vi "Purge.vi"(5 "Digital I/O Pin":u8=7, 7 "Arduino Resource":T1={"VISA resource"="GlueCTRL", "Board Type"=enum."Uno", "Connection Type"=enum."USB / Serial", "Bytes Per Packet (15)"=15}, 8 "Purge Time [ms]":dbl format="%#_13g", 9 "Axis Speeds":T3={"X [mm/s]"=25.0, "Y [mm/s]"=25.0, "Z [mm/s]"=25.0}, 10 "Start Position [mm]":dbl[](array[numeric]), 11 ".NET Refnum In":refnum<k24>) -> ()   [LabVIEW 2016]
uses:
  C:/Users/Aerotech/Documents/BNLStaveAssembly-blueprint/Bin/Aerotech.A3200.dll
  BNLStaveAssembly-blueprint/Bin/Aerotech.A3200.dll
  <vilib>/LabVIEW Interface for Arduino/Type Defs/Arduino Resource.ctl
  <vilib>/LabVIEW Interface for Arduino/Type Defs/Board Type.ctl
  <vilib>/LabVIEW Interface for Arduino/LabVIEW Interface for Arduino.lvlib
panel:
  in  "Change to Purge [mm]":dbl[](array[numeric])=[0.0, -15.0, 0.0]
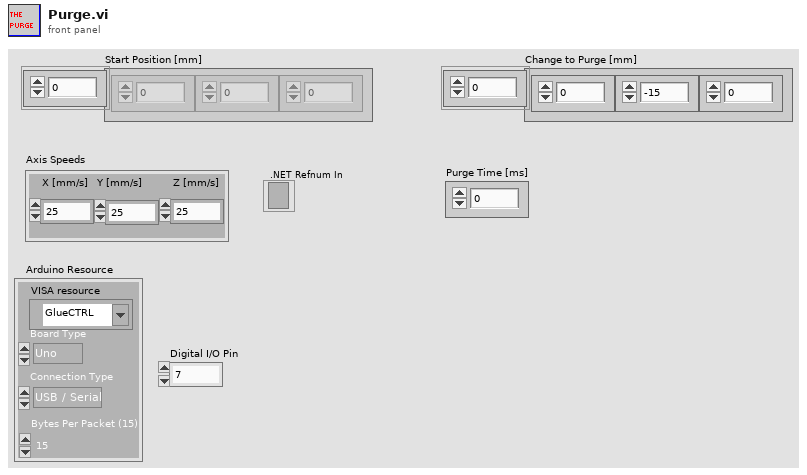
[diagram p1: front panel]
types:
  T1 = typedef "LabVIEW Interface for Arduino.lvlib/Arduino Resource.ctl" = cluster{"VISA resource":refnum<visa-resource-name>, "Board Type":T2, "Connection Type":enum8{"USB / Serial"}, "Bytes Per Packet (15)":u8}
  T2 = typedef "LabVIEW Interface for Arduino.lvlib/Board Type.ctl" = enum16{"Uno", "Dimuelanove w/Atmega 328", "Mega 2560"}
  T3 = cluster{"X [mm/s]":dbl, "Y [mm/s]":dbl, "Z [mm/s]":dbl}
  T4 = cluster{"Start Position [mm][0]":dbl, "Start Position [mm][1]":dbl, "Start Position [mm][2]":dbl}
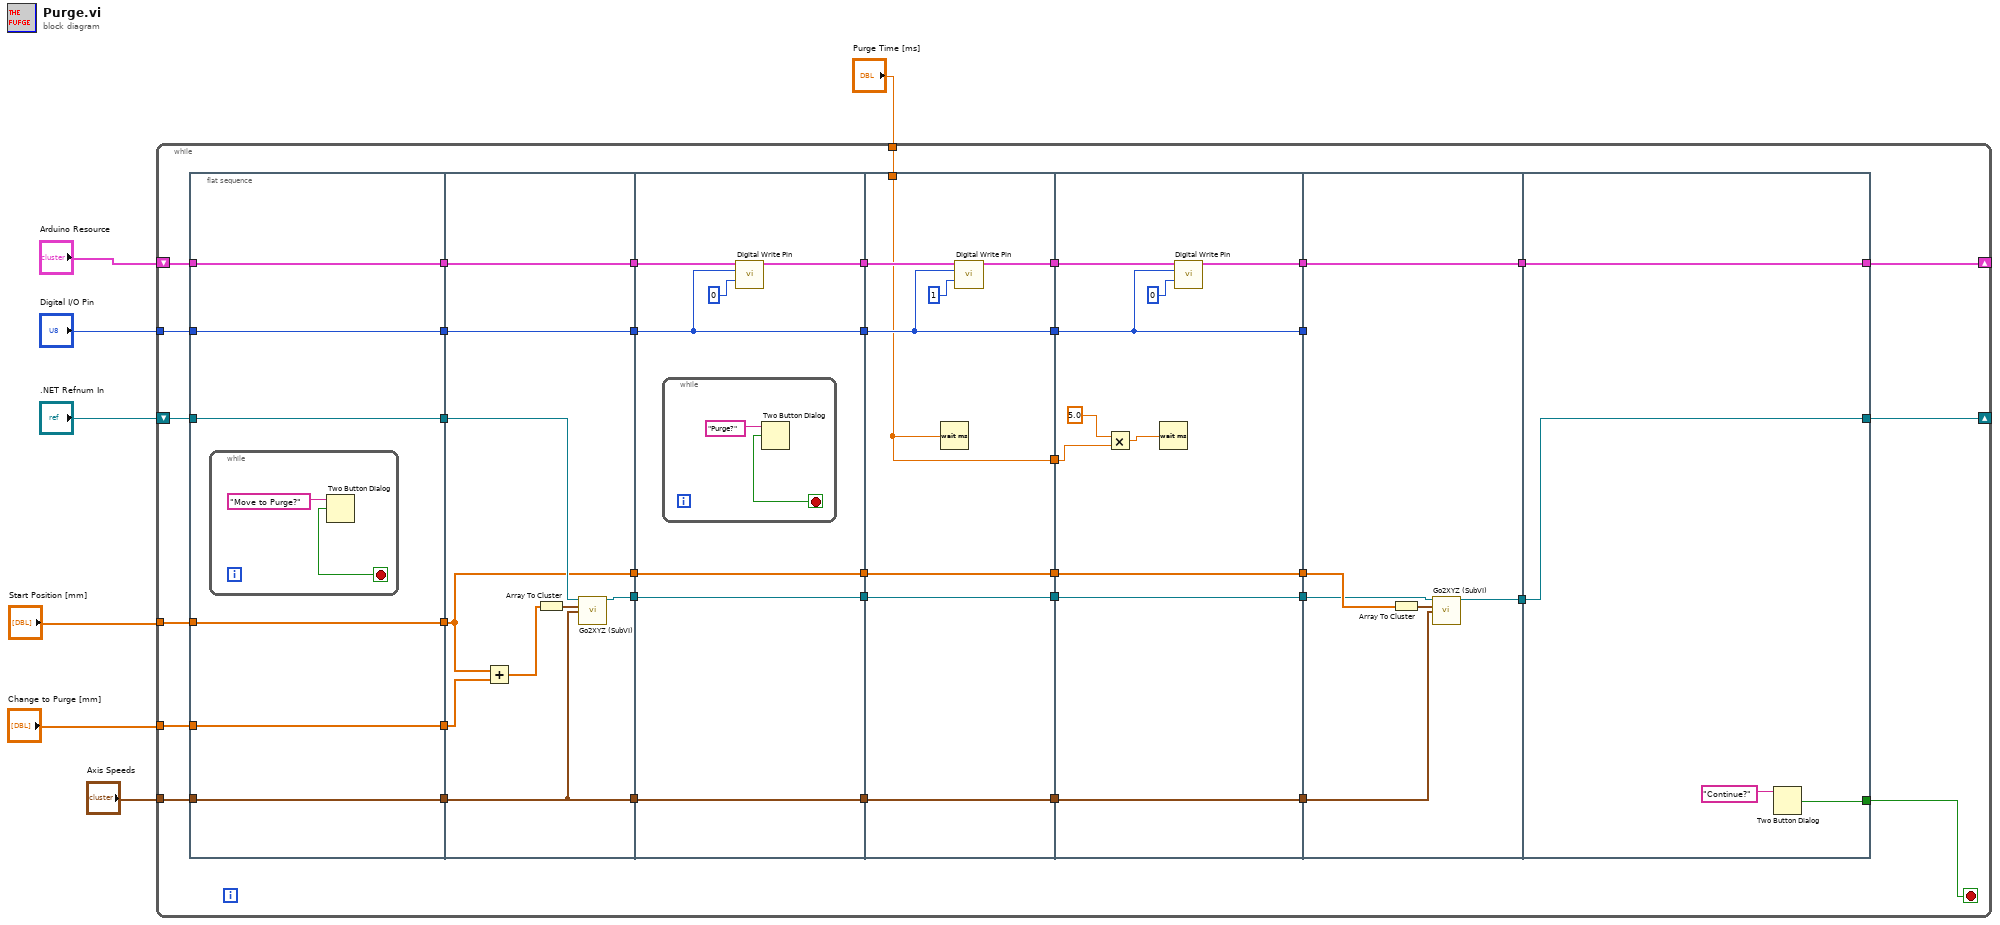
[diagram p0: block diagram]
diagram:
  n1 = while {
    tunnel: "Start Position [mm]" -> [w44]
    tunnel: "Change to Purge [mm]" -> [w43]
    tunnel: "Axis Speeds" -> [w40]
    shift-right: [w30] -> _
    shift-left: ".NET Refnum In" -> [w35]
    tunnel: "Digital I/O Pin" -> [w26]
    shift-right: [w13] -> _
    shift-left: "Arduino Resource" -> [w28]
    tunnel: "Purge Time [ms]" -> [w9]
    stop <- w46 stop-if-true
    n2 = flat-sequence {
      tunnel: [w52] -> w45
      tunnel: w44 -> [w52]
      tunnel: w43 -> [w51]
      tunnel: [w51] -> w42
      tunnel: [w50] -> w41
      tunnel: w40 -> [w50]
      tunnel: [w49] -> w39
      tunnel: w35 -> [w49]
      tunnel: [w48] -> w29
      tunnel: w28 -> [w48]
      tunnel: w26 -> [w47]
      tunnel: [w47] -> w25
      tunnel: w45 -> [w59]
      tunnel: w42 -> [w63]
      tunnel: w41 -> [w57]
      tunnel: w39 -> [w60]
      tunnel: [w59] -> w38
      tunnel: [w58] -> w37
      tunnel: [w57] -> w36
      tunnel: w29 -> [w56]
      tunnel: [w56] -> w27
      tunnel: w25 -> [w55]
      tunnel: [w55] -> w24
      tunnel: [w70] -> w23
      tunnel: w38 -> [w70]
      tunnel: [w69] -> w21
      tunnel: w37 -> [w69]
      tunnel: [w68] -> w19
      tunnel: w36 -> [w68]
      tunnel: w27 -> [w66]
      tunnel: w24 -> [w64]
      tunnel: [w65] -> w17
      tunnel: [w64] -> w11
      tunnel: w23 -> [w80]
      tunnel: [w80] -> w22
      tunnel: w21 -> [w79]
      tunnel: [w79] -> w20
      tunnel: w19 -> [w78]
      tunnel: [w78] -> w18
      tunnel: w17 -> [w76]
      tunnel: [w75] -> w16
      tunnel: [w74] -> w12
      tunnel: w11 -> [w74]
      tunnel: w9 -> [w73]
      tunnel: [w73] -> w8
      tunnel: w22 -> [w90]
      tunnel: [w90] -> w33
      tunnel: w20 -> [w89]
      tunnel: [w89] -> w32
      tunnel: w18 -> [w88]
      tunnel: [w88] -> w31
      tunnel: w16 -> [w86]
      tunnel: [w85] -> w14
      tunnel: w12 -> [w84]
      tunnel: [w84] -> w10
      tunnel: w8 -> [w82]
      tunnel: w33 -> [w96]
      tunnel: w32 -> [w94]
      tunnel: w31 -> [w93]
      tunnel: [w92] -> w34
      tunnel: [w91] -> w15
      tunnel: w14 -> [w91]
      tunnel: w10 -> [_]
      tunnel: [w99] -> w46
      tunnel: w34 -> [w98]
      tunnel: [w98] -> w30
      tunnel: [w97] -> w13
      tunnel: w15 -> [w97]
      frame #0 {
        n3 = while {
          stop <- w53 stop-if-true
          n4 = Two Button Dialog(message="Move to Purge?") -> (T button?=w53:bool)  [unwired: 2 in]
        }
      }
      frame #1 {
        n5 = Add(x=w59, y=w63) -> (x+y=w62:dbl[])
        n6 = Array To Cluster(array=w62) -> (cluster=w61:cluster{"[0]":dbl, "[1]":dbl, "[2]":dbl})
        n7 = call "Go2XYZ (SubVI).vi"(".NET Refnum in"=w60, "Go to Coordinates"=w61, "Axis Speeds"=w57) -> (".NET Refnum out"=w58:refnum<k24>)  [unwired: 8 in, 4 out]
      }
      frame #2 {
        n8 = while {
          stop <- w71 stop-if-true
          n9 = Two Button Dialog(message="Purge?") -> (T button?=w71:bool)  [unwired: 2 in]
        }
        n10 = call <vilib>:"Digital Write Pin.vi"("Arduino Resource"=w66, "Digital I/O Pin (0)"=w64, "Value (0)"=u8 0) -> ("Arduino Resource"=w65:T1)  [unwired: 11 in, 1 out]
      }
      frame #3 {
        n11 = Wait (ms)(milliseconds to wait=w73) -> ()  [unwired: 1 out]
        n12 = call <vilib>:"Digital Write Pin.vi"("Arduino Resource"=w76, "Digital I/O Pin (0)"=w74, "Value (0)"=u8 1) -> ("Arduino Resource"=w75:T1)  [unwired: 11 in, 1 out]
      }
      frame #4 {
        n13 = Multiply(x=5.0, y=w82) -> (x*y=w83:dbl)
        n14 = Wait (ms)(milliseconds to wait=w83) -> ()  [unwired: 1 out]
        n15 = call <vilib>:"Digital Write Pin.vi"("Arduino Resource"=w86, "Digital I/O Pin (0)"=w84, "Value (0)"=u8 0) -> ("Arduino Resource"=w85:T1)  [unwired: 11 in, 1 out]
      }
      frame #5 {
        n16 = Array To Cluster(array=w96) -> (cluster=w95:T4)
        n17 = call "Go2XYZ (SubVI).vi"(".NET Refnum in"=w94, "Go to Coordinates"=w95, "Axis Speeds"=w93) -> (".NET Refnum out"=w92:refnum<k24>)  [unwired: 8 in, 4 out]
      }
      frame #6 {
        n18 = Two Button Dialog(message="Continue?") -> (T button?=w99:bool)  [unwired: 2 in]
      }
    }
  }
